vi "5492_AutonomousMotor.vi"(9 "Length":dbl=3000.0, 10 "Position Goal":dbl) -> (2 "Done":bool)   [LabVIEW 2017]
uses:
  5492_WPI_RobotDriveMotorSelectorEnum.ctl
  Public/Documents/Cross The Road Electronics/Phoenix-LabVIEW/Motor Controller/Controls/CTRE_Phoenix_MotorControl_ControlMode.ctl
  <vilib>/Rock Robotics/WPI/Utilities/WPI_GetSetVariantRefNum.vi
  <vilib>/Rock Robotics/WPI/RobotDrive/WPI_RobotDriveSafetyCheck.vi
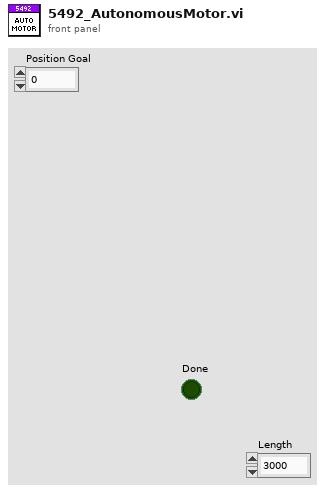
[diagram p1: front panel]
types:
  T1 = typedef "5492_WPI_RobotDriveMotorSelectorEnum.ctl" = enum16{"Front left motor", "Front right motor"}
  T2 = typedef "WPI_RobotDriveDevRef.ctl" = cluster{"DevStatus":errorcluster, "Motors[]":T3[], "Square Inputs":bool, "Max Output":dbl}
  T3 = typedef "WPI_MotorControlDeviceRef.ctl" = cluster{"DeviceStatus":errorcluster, "Type":T4, "PWM":cluster{"PWM Channel":T5, "DeadBand":T6}, "CAN":cluster{"Device Number":u8, "SetOutput VI Ref":variant, "GetOutput VI Ref":variant, "Enable VI Ref":variant, "Disable VI Ref":variant, "Data":variant}, "Invert":bool, "DIO PWM":cluster{"PWM \"Enable\" Channel":T5, "DIOChannel":T7, "PWM Rate":dbl}}
  T4 = typedef "WPI_MotorControlType.ctl" = enum16{"PWM", "CAN", "DIO PWM"}
  T5 = typedef "FPGA_DIOPWMChannel.ctl" = enum8{"PWM 0", "PWM 1", "PWM 2", "PWM 3", "PWM 4", "PWM 5", "PWM 6", "PWM 7", "PWM 8", "PWM 9", "PWM MXP 0", "PWM MXP 1", "PWM MXP 2", "PWM MXP 3", "PWM MXP 4", "PWM MXP 5", "PWM MXP 6", "PWM MXP 7", "PWM MXP 8", "PWM MXP 9", "Invalid"}
  T6 = typedef "WPI_PWMDeadband.ctl" = cluster{"Name":string, "maxPositivePwm":i32, "minPositivePwm":i32, "centerPwm":i32, "maxNegativePwm":i32, "minNegativePwm":i32, "angularRange":u16}
  T7 = typedef "FPGA_DIOChannel.ctl" = enum8{"DIO 0", "DIO 1", "DIO 2", "DIO 3", "DIO 4", "DIO 5", "DIO 6", "DIO 7", "DIO 8", "DIO 9", "DIO MXP 0", "DIO MXP 1", "DIO MXP 2", "DIO MXP 3", "DIO MXP 4", "DIO MXP 5", "DIO MXP 6", "DIO MXP 7", "DIO MXP 8", "DIO MXP 9", "DIO MXP 10", "DIO MXP 11", "DIO MXP 12", "DIO MXP 13", "DIO MXP 14", "DIO MXP 15", "SPI Port CS1", "SPI Port CS2", "SPI Port CS3", "SPI Port MISO", "SPI Port MOSI", "Invalid"}
  T8 = typedef "CTRE_Phoenix_MotorControl_ControlMode.ctl" = u16
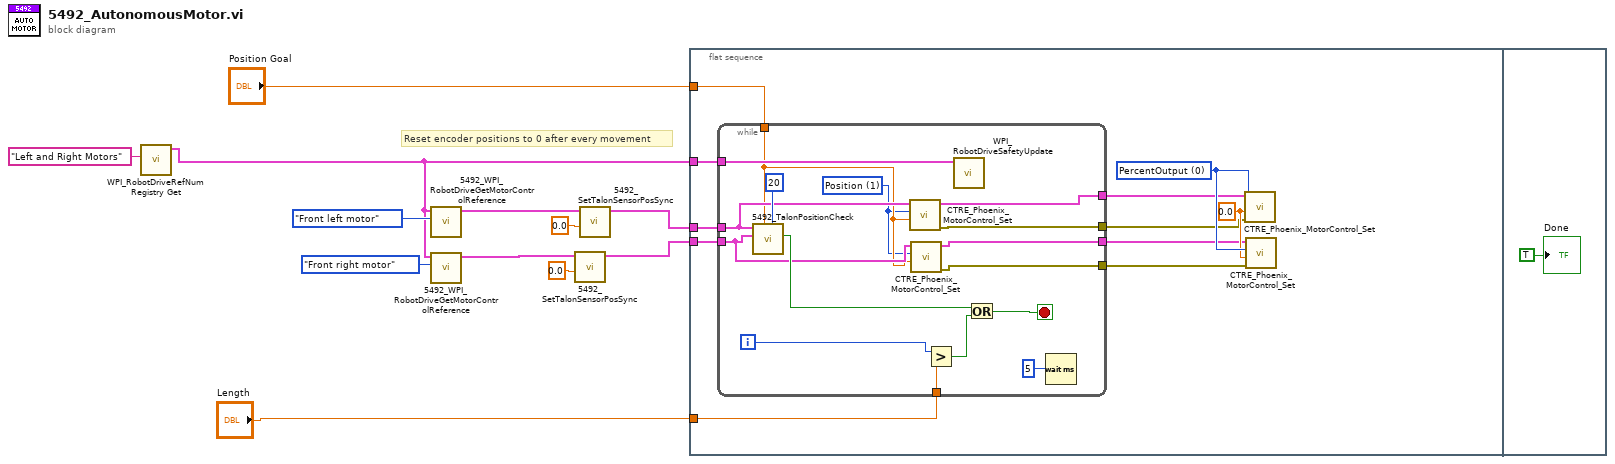
[diagram p0: block diagram]
diagram:
  # "Reset encoder positions to 0 after every movement"
  n1 = call <vilib>:"WPI_RobotDriveRefNum Registry Get.vi"("refnum name"="Left and Right Motors") -> ("RobotDriveDevRef"=w1:T2)  [unwired: 9 in, 1 out]
  n2 = call "5492_WPI_RobotDriveGetMotorControlReference.vi"("MotorIndex"=5492_WPI_RobotDriveMotorSelectorEnum."Front left motor", "RobotDriveDevRef"=w1) -> ("MotorControlDeviceRef"=w9:T3)  [unwired: 9 out]
  n3 = call "5492_WPI_RobotDriveGetMotorControlReference.vi"("MotorIndex"=5492_WPI_RobotDriveMotorSelectorEnum."Front right motor", "RobotDriveDevRef"=w1) -> ("MotorControlDeviceRef"=w7:T3)  [unwired: 9 out]
  n4 = call "5492_SetTalonSensorPosSync.vi"("Pos"=0.0 ("New Sensor Position"), "CAN Talon SRX Ref In"=w7) -> ("CAN Talon SRX Ref Out"=w6:T3)  [unwired: 8 in, 1 out]
  n5 = call "5492_SetTalonSensorPosSync.vi"("Pos"=0.0 ("New Sensor Position"), "CAN Talon SRX Ref In"=w9) -> ("CAN Talon SRX Ref Out"=w5:T3)  [unwired: 8 in, 1 out]
  n6 = flat-sequence {
    tunnel: w6 -> [w23]
    tunnel: w5 -> [w22]
    tunnel: "Length" -> [w21]
    tunnel: "Position Goal" -> [w20]
    tunnel: w1 -> [w19]
    frame #0 {
      w18 = T8 0 items=["PercentOutput"=0, "Position"=1, "Velocity"=2, "Current"=3, "Follower"=5, "MotionProfile"=6, "MotionMagic"=7, "MotionMagicArc"=8, "MotionProfileArc"=10, "Disabled"=15] ("Control Mode")
      w17 = 0.0 ("Output")
      n7 = while {
        tunnel: w23 -> [w30]
        tunnel: w22 -> [w31]
        tunnel: w21 -> [w35]
        tunnel: w20 -> [w29]
        tunnel: w19 -> [w32]
        tunnel: [w27] -> w16
        tunnel: [w26] -> w15
        tunnel: [w25] -> w14
        tunnel: [w24] -> w13
        i -> [w36]
        stop <- w39 stop-if-true
        w28 = T8 1 items=["PercentOutput"=0, "Position"=1, "Velocity"=2, "Current"=3, "Follower"=5, "MotionProfile"=6, "MotionMagic"=7, "MotionMagicArc"=8, "MotionProfileArc"=10, "Disabled"=15] ("Control Mode")
        n8 = call "5492_TalonPositionCheck.vi"("Margin of Error"=20, "Position Goal"=w29, "CAN Talon SRX Ref Right"=w30, "CAN Talon SRX Ref Left"=w31) -> ("Goal Achieved"=w38:bool)  [unwired: 7 in]
        n9 = call "CTRE_Phoenix_MotorControl_Set.vi"("Output"=w29, "Control Mode"=w28, "PhoenixMotorControlDevRef"=w31) -> ("error out"=w25:errorcluster, "PhoenixMotorControlDevRef"=w27:T3)  [unwired: 7 in]
        n10 = call "CTRE_Phoenix_MotorControl_Set.vi"("Output"=w29, "Control Mode"=w28, "PhoenixMotorControlDevRef"=w30) -> ("error out"=w24:errorcluster, "PhoenixMotorControlDevRef"=w26:T3)  [unwired: 7 in]
        n11 = Greater?(x=w36, y=w35) -> (0:w37:bool)
        n12 = call <vilib>:"WPI_RobotDriveSafetyUpdate.vi"("RobotDriveDevRef"=w32) -> ()  [unwired: 1 in, 10 out]
        n13 = Or(x=w38, y=w37) -> (x .or. y?=w39:bool)
        n14 = Wait (ms)(milliseconds to wait=u32 5) -> ()  [unwired: 1 out]
      }
      n15 = call "CTRE_Phoenix_MotorControl_Set.vi"("error in (no error)"=w14, "Output"=w17, "Control Mode"=w18, "PhoenixMotorControlDevRef"=w16) -> ()  [unwired: 6 in, 2 out]
      n16 = call "CTRE_Phoenix_MotorControl_Set.vi"("error in (no error)"=w13, "Output"=w17, "Control Mode"=w18, "PhoenixMotorControlDevRef"=w15) -> ()  [unwired: 6 in, 2 out]
    }
    frame #1 {
      "Done" <- TRUE ("Done")
    }
  }
